vi "Verify with Regex Scrubber.vi"(8 "error in":errorcluster) -> (0 "error out":errorcluster)   [LabVIEW 2020, in "Caraya Extension Tests.lvclass"]
uses:
  Caraya Extension Tests.lvclass
  Source/Approval Tests/Options.ctl
  Source/Approval Tests/Reporter/Reporter.lvclass
  Source/Approval Tests/Namer/Namer.lvclass
  Source/Approval Tests/Scrubber/Scrubber.lvclass
  Source/Approval Tests/Regex Scrubber/Regex Scrubber.lvclass
  C:/Users/SAS/Desktop/ApprovalTests.LabVIEW/Source/Approval Tests/Scrubber/Scrubber.lvclass
  Source/Approval Tests/Regex Scrubber/Regex Scrubber.lvclass/Regex Scrubber.ctl
  4b862e9e-fcb2-487f-ab73-d9f83fbf4d2c.vi
  Source/Approval Tests/Regex Scrubber/Write Regex.vi
  Source/Approval Tests/Regex Scrubber/Write Replacement.vi
  4b862e9e-fcb2-487f-ab73-d9f83fbf4d2c.vi/500b534b-d6f0-4fa5-90b2-c40158375321.vi
  4b862e9e-fcb2-487f-ab73-d9f83fbf4d2c.vi/500b534b-d6f0-4fa5-90b2-c40158375321.vi/93c5622b-9fb7-41e0-8c76-3fde37e94e34.vi
  4b862e9e-fcb2-487f-ab73-d9f83fbf4d2c.vi/500b534b-d6f0-4fa5-90b2-c40158375321.vi/93c5622b-9fb7-41e0-8c76-3fde37e94e34.vi/daceb942-e4a5-48f9-868a-a7549e7f6e2f.vi
  Source/Approval Tests/Replace with Caller if Empty.vi
  Source/Approval Tests/conv EOL.vi
  <vilib>/Utility/libraryn.llb/Check if File or Folder Exists.vi
  <vilib>/addons/_JKI Toolkits/Caraya/classes/Assert/Assert.vi
  <vilib>/addons/_JKI Toolkits/Caraya/classes/Assert/Assert True.vi
  <vilib>/addons/_JKI Toolkits/Caraya/classes/Test/Test.lvclass
  Source/Approval Tests/Approval Tests.lvlib
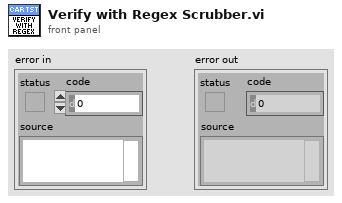
[diagram p1: front panel]
types:
  T1 = typedef "Approval Tests.lvlib/Options.ctl" = cluster{"Reporter":refnum<class "Reporter.lvclass">, "Extension(txt)":string, "Namer":refnum<class "Namer.lvclass">, "Scrubber":refnum<class "Scrubber.lvclass">, "Test Label":string}
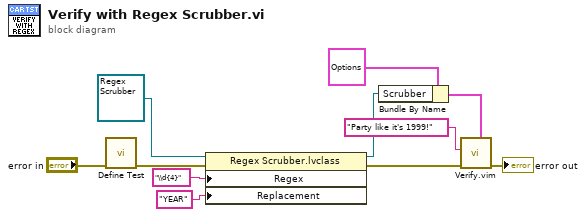
[diagram p0: block diagram]
diagram:
  n1 = call <vilib>:"Define Test.vi"("error in (no error)"="error in") -> ("error out"=w11:errorcluster)  [unwired: 9 in, 1 out]
  n2 = property class="Regex Scrubber.lvclass"(reference=refnum<class "Regex Scrubber.lvclass"> refnum ("Approval Tests.lvlib:Regex Scrubber.lvclass"), error in=w11, "Regex"="\\d{4}", "Replacement"="YEAR") -> (reference out=w4:refnum<class "Regex Scrubber.lvclass">, error out=w8:errorcluster)
  n3 = Bundle By Name(cluster=T1 {"Reporter"=refnum, "Extension(txt)"="", "Namer"=refnum, "Scrubber"=refnum, "Test Label"=""} ("Options"), "Scrubber"=w4) -> (w5:T1)
  n4 = call "Verify.vim"("Options"=w5, "error in"=w8, "Test Data"="Party like it's 1999!") -> ("error out"=→"error out":errorcluster)  [unwired: 8 in]
